vi "HumiditySensorInput.vi"(0 "FPGA I/O In":refnum<k21>="ConnectorA/DIO4") -> (4 "Temperature (°C)":fxp<+,16,7> format="%.11g", 6 "Humidity (%)":fxp<+/-,18,8> format="%.12g", 15 "error out":errorcluster)   [LabVIEW 2015, in "DHT22 (FPGA).lvlib"]
doc: "Read Temperature and Humidity from DHT11 Sensor.\n\n\nError Codes\n========\n\nError -8001: Checksum Error\nError- 8002: Timeout Error"
uses:
  DHT22 (FPGA).lvlib
  Command.ctl
  <vilib>/Platform/TimedLoop/XDataNode/timing_clust.ctl
  <vilib>/Platform/TimedLoop/XDataNode/nitl_modes.ctl
  <vilib>/Platform/TimedLoop/XDataNode/wakeup.ctl
  <vilib>/rvi/Emulation/niFpgaGetClockAttributes.vi
  <vilib>/rvi/Emulation/niFpgaSctlEmulationGetInTimedLoop.vi
  <vilib>/rvi/Emulation/niFpgaEmulationReportErrorSimple.vi
  <vilib>/rvi/Emulation/niFpgaProcessEmulError.vi
  <vilib>/rvi/Emulation/niFpgaCriticalErrorInLSC.vi
  <vilib>/rvi/eio/common/nirviEmuTemplateMethod_errors.vi
  <vilib>/Platform/TimedLoop/XDataNode/XDataNode.xnode
  <vilib>/eio/EIOMethodNode/EIOMethodNode.xnode
  <vilib>/eio/EIONode/EIONode.xnode
  <vilib>/Platform/TimedLoop/XDataNode/XDNodeRunTimeDep.lvlib
panel:
  in  "STOP Reading Inputs":bool
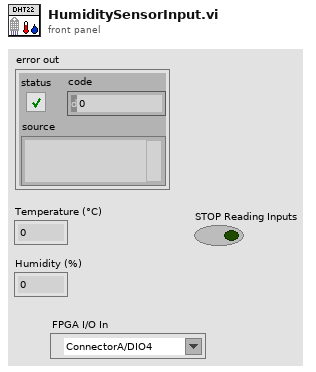
[diagram p1: front panel]
types:
  T1 = typedef "DHT22 (FPGA).lvlib/Command.ctl" = enum16{"Send Start Signal", "Wait Low", "Host Pulls Up", "Wait High", "Change to Read", "Wait for Sensor Response Signal Low", "Wait for Sensor Response Signal High", "Start Data Transmission", "Read Data", "Scale and Checksum", "Checksum Error", "Timeout Error"}
  T2 = typedef "XDNodeRunTimeDep.lvlib/timing_clust.ctl" = cluster{"Expected End [f-1]":u64, "Actual End [f-1]":u64, "Finished Late? [f-1]":bool, "Expected End [i-1]":u64, "Actual End [i-1]":u64, "Finished Late? [i-1]":bool, "Expected Start [i]":u64, "Actual Start [i]":u64, "Expected Start [f]":u64, "Actual Start [f]":u64, "Source Name":string, "Structure Name":string, "Period":i64, "Deadline":i64, "Offset":i64, "Start":i64, "Priority":i32, "Timeout":i32, "Mode":T3, "Wakeup Reason":T4, "Error":errorcluster, "Source Type":string, "Secondary Source Type":string, "Global End Time":u64, "Global Start Time":u64, "Frame Duration":u64, "Iteration Duration":u64, "Assigned CPU":i32, "I/O Scan Engine Mode":u32}
  T3 = typedef "XDNodeRunTimeDep.lvlib/nitl_modes.ctl" = enum32{"No Change", "Process missed periods, maintain original phase", "Discard missed periods, maintain original phase", "Process missed periods, ignore original phase", "Discard missed periods, ignore original phase"}
  T4 = typedef "XDNodeRunTimeDep.lvlib/wakeup.ctl" = enum32{"Normal", "Aborted", "Asynchronous wakeup", "Timing source error", "Timed loop error", "Timeout"}
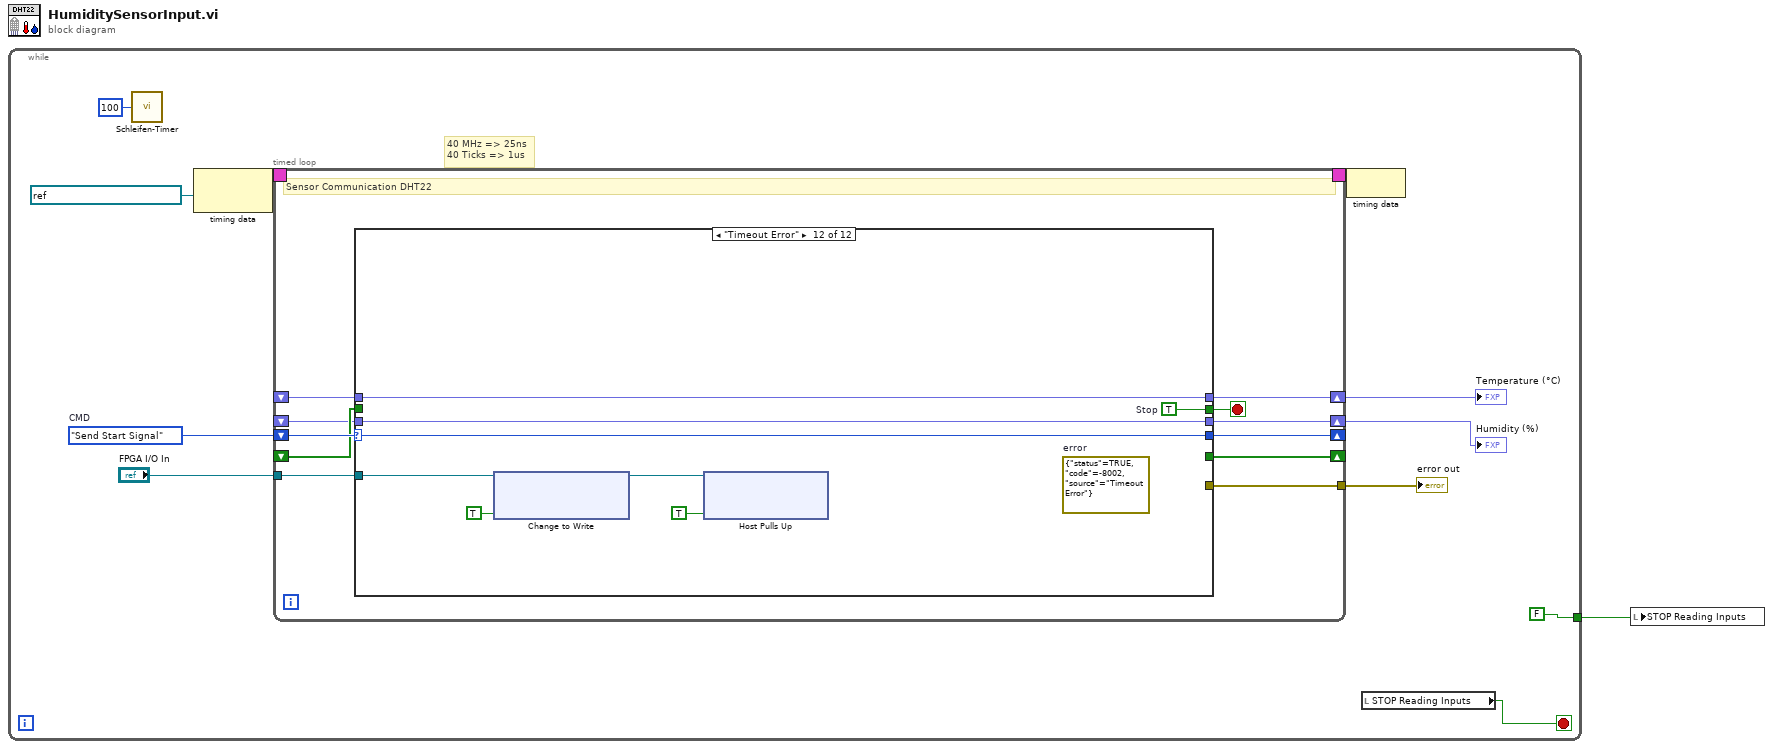
[diagram p0: block diagram]
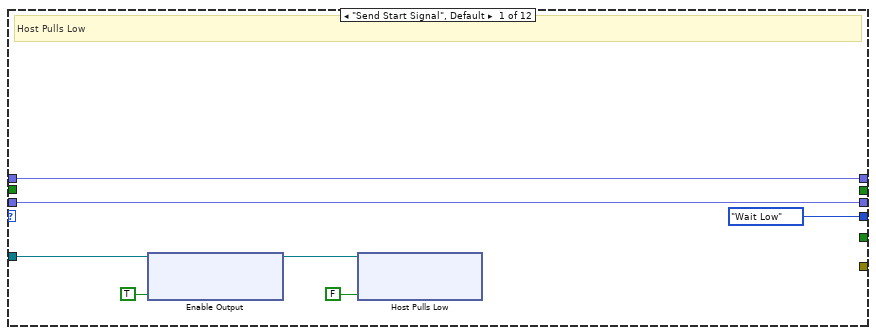
[diagram p2: hidden frame]
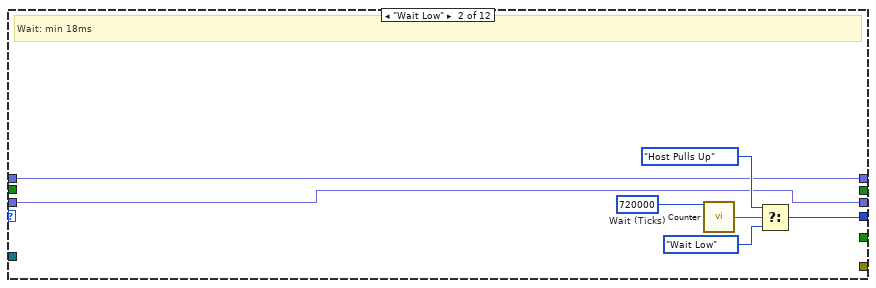
[diagram p3: hidden frame]
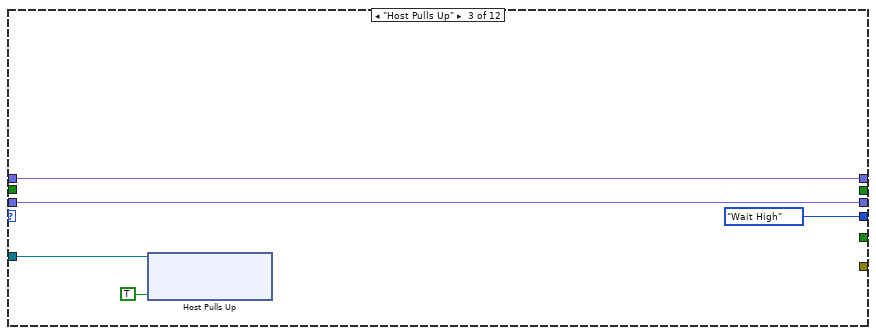
[diagram p4: hidden frame]
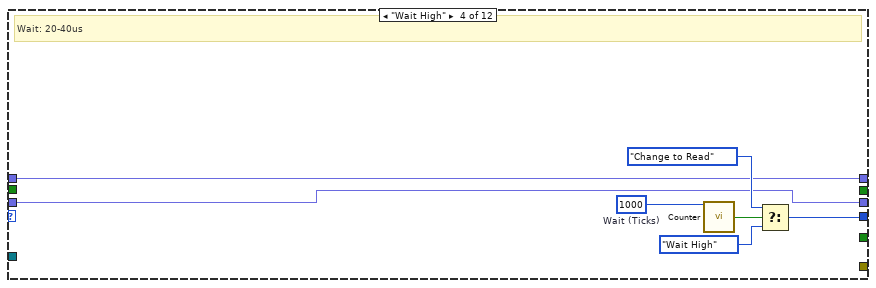
[diagram p5: hidden frame]
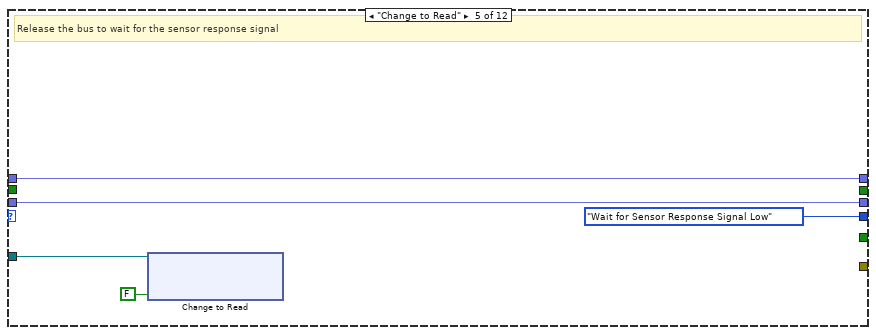
[diagram p6: hidden frame]
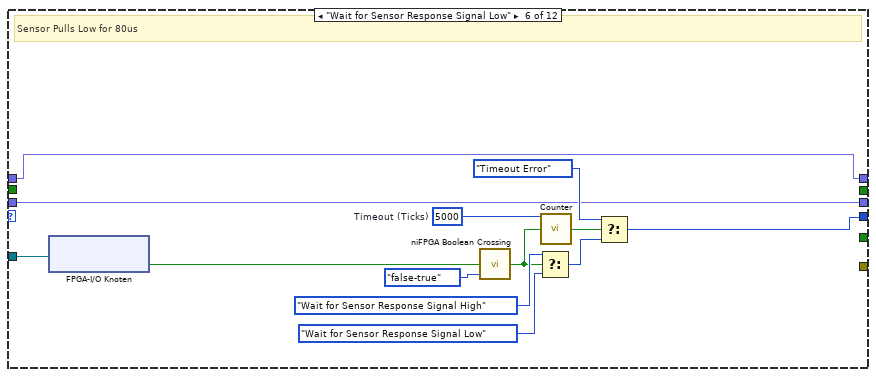
[diagram p7: hidden frame]
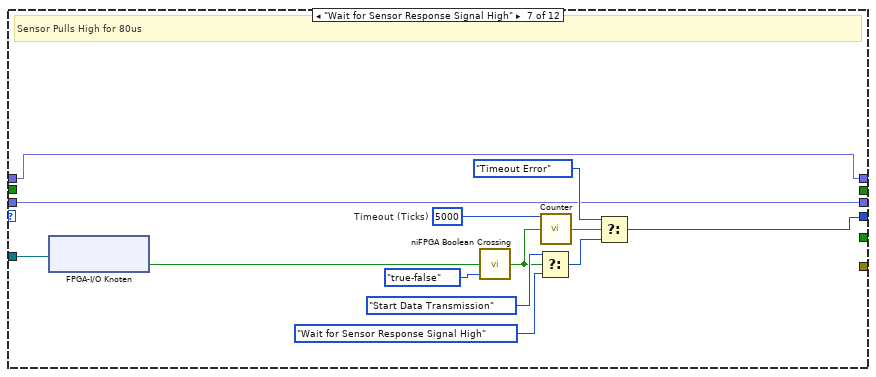
[diagram p8: hidden frame]
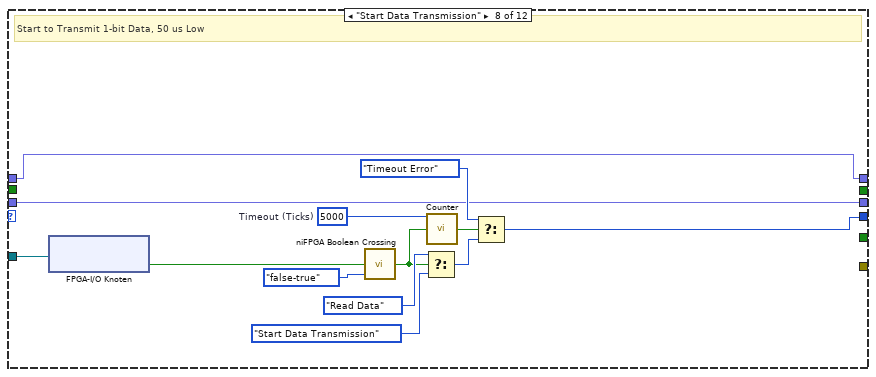
[diagram p9: hidden frame]
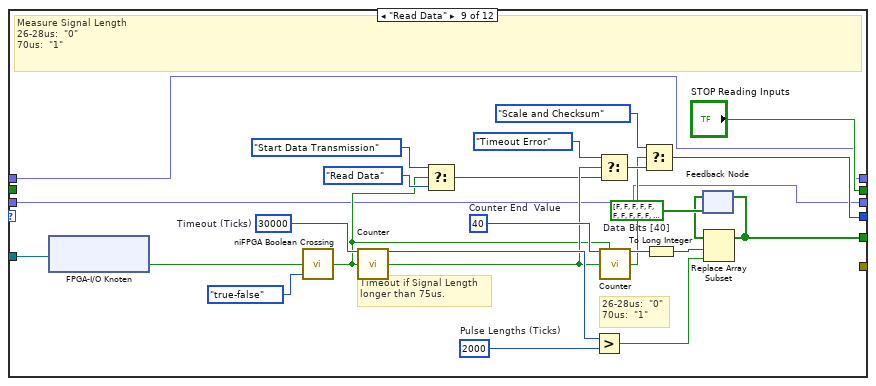
[diagram p10: hidden frame]
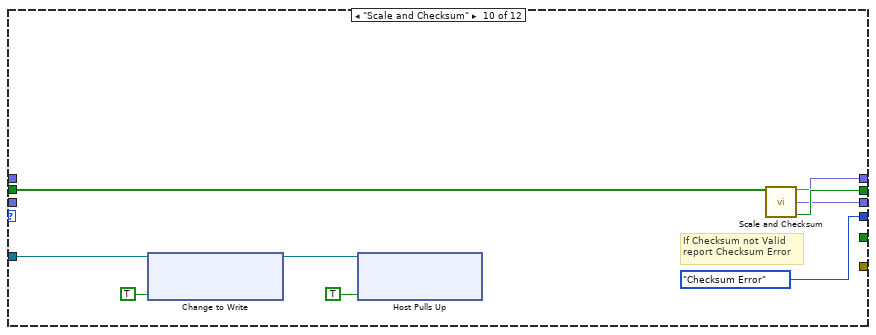
[diagram p11: hidden frame]
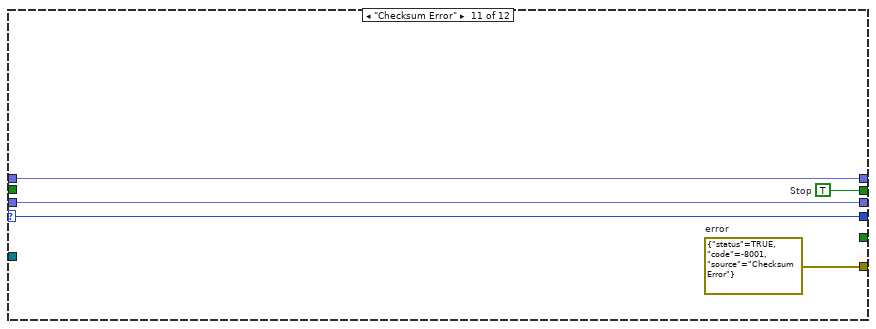
[diagram p12: hidden frame]
diagram:
  n1 = while {
    tunnel: [FALSE] -> w1
    stop <- w3 stop-if-true
    w10 = Command."Send Start Signal"  # CMD
    # "40 MHz => 25ns\n40 Ticks => 1us"
    n2 = call "Schleifen-Timer"("Count(mSec)"=u32 100) -> ()  [unwired: 1 out]
    n3 = node-c288(refnum<k21> "40 MHz Onboard Clock" ("Source Name")) -> (w12:T2)
    n4 = timed-loop {
      timing: w12 -> [_]
      timing-out: [_] -> w11
      shift-right: [w21] -> _
      shift-left: w10 -> [w23]
      tunnel: "FPGA I/O In" -> [w22]
      shift-right: [w19] -> _
      shift-left: _ -> [w18]
      tunnel: [w15] -> w6
      shift-right: [w17] -> w8
      shift-left: _ -> [w14]
      shift-right: [w16] -> w7
      shift-left: _ -> [w13]
      stop <- w20 stop-if-true
      # "Sensor Communication DHT22"
      n5 = case shown="\"Timeout Error\"" w23 {
        selector: w23 -> [_ _ _ _ _ _ _ _ _ _ w132 w140]
        tunnel: w22 -> [w29 _ w41 _ w53 w67 w80 w93 w119 w125 _ w136]
        tunnel: [Command."Wait Low" ("CMD") w35 Command."Wait High" ("CMD") w45 Command."Wait for Sensor Response Signal Low" ("CMD") w61 w74 w87 w100 Command."Checksum Error" ("CMD") w132 w140] -> w21
        tunnel: [_ _ _ _ _ _ _ _ "STOP Reading Inputs" w123 w133 w141] -> w20
        tunnel: [_ _ _ _ _ _ _ _ w98 _ _ _] -> w19
        tunnel: w18 -> [_ _ _ _ _ _ _ _ _ w124 _ _]
        tunnel: [w25 w31 w38 w43 w50 w55 w68 w81 w94 w121 w129 w134] -> w17
        tunnel: [w24 w32 w39 w44 w51 w56 w69 w82 w95 w120 w130 w135] -> w16
        tunnel: [_ _ _ _ _ _ _ _ _ _ w131 _] -> w15
        tunnel: w14 -> [w25 w31 w38 w43 w50 w55 w68 w81 w94 _ w129 w134]
        tunnel: w13 -> [w24 w32 w39 w44 w51 w56 w69 w82 w95 _ w130 w135]
        frame "Send Start Signal", Default {
          # "Host Pulls Low"
          n6 = xnode "Enable Output"("FPGA I/O In"=w29, "Enable"=TRUE ("Data")) -> ("FPGA I/O Out"=w27:refnum<k21>)
          n7 = xnode "Host Pulls Low"("FPGA I/O In"=w27, "Data"=FALSE ("Enable")) -> ()  [unwired: 1 out]
        }
        frame "Wait Low" {
          w37 = u32 720000  # Wait (Ticks)
          # "Wait: min 18ms"
          n8 = call "Counter.vi"("Counter End  Value"=w37) -> ("End Reached"=w33:bool)  [unwired: 13 in, 1 out]
          n9 = Select(t=Command."Host Pulls Up" ("CMD"), s=w33, f=Command."Wait Low" ("CMD")) -> (s? t:f=w35:T1)
        }
        frame "Host Pulls Up" {
          n10 = xnode "Host Pulls Up"("FPGA I/O In"=w41, "Data"=TRUE ("Enable")) -> ()  [unwired: 1 out]
        }
        frame "Wait High" {
          w49 = u32 1000  # Wait (Ticks)
          # "Wait: 20-40us"
          n11 = call "Counter.vi"("Counter End  Value"=w49) -> ("End Reached"=w46:bool)  [unwired: 13 in, 1 out]
          n12 = Select(t=Command."Change to Read" ("CMD"), s=w46, f=Command."Wait High" ("CMD")) -> (s? t:f=w45:T1)
        }
        frame "Change to Read" {
          # "Release the bus to wait for the sensor response signal"
          n13 = xnode "Change to Read"("FPGA I/O In"=w53, "Enable"=FALSE ("Data")) -> ()  [unwired: 1 out]
        }
        frame "Wait for Sensor Response Signal Low" {
          w66 = u32 5000  # Timeout (Ticks)
          # "Sensor Pulls Low for 80us"
          n14 = xnode "FPGA-I/O Knoten"("FPGA-I/O (Eingang)"=w67) -> ("I/O-Objekt"=w62:bool)  [unwired: 1 out]
          n15 = call <vilib>:"niFPGA Boolean Crossing.vi"("input"=w62, "direction"=enum8{"either", "false-true", "true-false"}."false-true") -> ("crossing"=w57:bool)  [unwired: 7 in]
          n16 = Select(t=Command."Wait for Sensor Response Signal High" ("CMD"), s=w57, f=Command."Wait for Sensor Response Signal Low" ("CMD")) -> (s? t:f=w60:T1)
          n17 = call "Counter.vi"("Counter End  Value"=w66, "Reset"=w57) -> ("End Reached"=w58:bool)  [unwired: 12 in, 1 out]
          n18 = Select(t=Command."Timeout Error", s=w58, f=w60) -> (s? t:f=w61:T1)
        }
        frame "Wait for Sensor Response Signal High" {
          w79 = u32 5000  # Timeout (Ticks)
          # "Sensor Pulls High for 80us"
          n19 = xnode "FPGA-I/O Knoten"("FPGA-I/O (Eingang)"=w80) -> ("I/O-Objekt"=w75:bool)  [unwired: 1 out]
          n20 = call <vilib>:"niFPGA Boolean Crossing.vi"("input"=w75, "direction"=enum8{"either", "false-true", "true-false"}."true-false") -> ("crossing"=w70:bool)  [unwired: 7 in]
          n21 = Select(t=Command."Start Data Transmission" ("CMD"), s=w70, f=Command."Wait for Sensor Response Signal High" ("CMD")) -> (s? t:f=w73:T1)
          n22 = call "Counter.vi"("Counter End  Value"=w79, "Reset"=w70) -> ("End Reached"=w71:bool)  [unwired: 12 in, 1 out]
          n23 = Select(t=Command."Timeout Error", s=w71, f=w73) -> (s? t:f=w74:T1)
        }
        frame "Start Data Transmission" {
          w92 = u32 5000  # Timeout (Ticks)
          # "Start to Transmit 1-bit Data, 50 us Low"
          n24 = xnode "FPGA-I/O Knoten"("FPGA-I/O (Eingang)"=w93) -> ("I/O-Objekt"=w88:bool)  [unwired: 1 out]
          n25 = call <vilib>:"niFPGA Boolean Crossing.vi"("input"=w88, "direction"=enum8{"either", "false-true", "true-false"}."false-true") -> ("crossing"=w83:bool)  [unwired: 7 in]
          n26 = Select(t=Command."Read Data" ("CMD"), s=w83, f=Command."Start Data Transmission" ("CMD")) -> (s? t:f=w86:T1)
          n27 = call "Counter.vi"("Counter End  Value"=w92, "Reset"=w83) -> ("End Reached"=w84:bool)  [unwired: 12 in, 1 out]
          n28 = Select(t=Command."Timeout Error", s=w84, f=w86) -> (s? t:f=w87:T1)
        }
        frame "Read Data" {
          w118 = u32 30000  # Timeout (Ticks)
          w112 = u32 2000  # Pulse Lengths (Ticks)
          w106 = u32 40  # Counter End  Value
          w110 = bool[] [FALSE, FALSE, FALSE, FALSE, FALSE, FALSE, FALSE, FALSE, FALSE, FALSE, FALSE, FALSE, FALSE, FALSE, FALSE, FALSE, FALSE, FALSE, FALSE, FALSE, FALSE, FALSE, FALSE, FALSE, FALSE, FALSE, FALSE, FALSE, FALSE, FALSE, FALSE, FALSE, FALSE, FALSE, FALSE, FALSE, FALSE, FALSE, FALSE, FALSE]  # Data Bits [40]
          # "26-28us:  \"0\"\n70us:  \"1\""
          # "Timeout if Signal Length\nlonger than 75us."
          # "Measure Signal Length\n26-28us:  \"0\"\n70us:  \"1\""
          n29 = xnode "FPGA-I/O Knoten"("FPGA-I/O (Eingang)"=w119) -> ("I/O-Objekt"=w114:bool)  [unwired: 1 out]
          n30 = call <vilib>:"niFPGA Boolean Crossing.vi"("input"=w114, "direction"=enum8{"either", "false-true", "true-false"}."true-false") -> ("crossing"=w103:bool)  [unwired: 7 in]
          n31 = call "Counter.vi"("Counter End  Value"=w118, "Reset"=w103) -> ("Counter Value"=w111:u32, "End Reached"=w104:bool)  [unwired: 12 in]
          n32 = Select(t=Command."Start Data Transmission" ("CMD"), s=w103, f=Command."Read Data" ("CMD")) -> (s? t:f=w102:T1)
          n33 = Greater?(x=w111, y=w112) -> (0:w107:bool)
          n34 = Select(t=Command."Timeout Error", s=w104, f=w102) -> (s? t:f=w99:T1)
          n35 = call "Counter.vi"("Counter End  Value"=w106, "Input Valid"=w103, "Reset"=w104) -> ("Counter Value"=w105:u32, "End Reached"=w97:bool)  [unwired: 11 in]
          n36 = Select(t=Command."Scale and Checksum", s=w97, f=w99) -> (s? t:f=w100:T1)
          n37 = To Long Integer(number=w105) -> (32bit integer=w108:i32)
          n38 = feedback #1(w110) -> (w109:bool[])
          n39 = Replace Array Subset(array=w109, new element=w107, index=w108) -> (w98:bool[])
          n40 = feedback-in #1(w98) -> ()
        }
        frame "Scale and Checksum" {
          # "If Checksum not Valid\nreport Checksum Error"
          n41 = xnode "Change to Write"("FPGA I/O In"=w125, "Enable"=TRUE ("Data")) -> ("FPGA I/O Out"=w126:refnum<k21>)
          n42 = xnode "Host Pulls Up"("FPGA I/O In"=w126, "Data"=TRUE ("Enable")) -> ()  [unwired: 1 out]
          n43 = call "Scale and Checksum.vi"("Raw Data"=w124) -> ("Temperature (°C)"=w121:fxp<+,16,7>, "Humidity (%)"=w120:fxp<+/-,18,8>, "Valid?"=w123:bool)  [unwired: 12 in]
        }
        frame "Checksum Error" {
          w131 = errorcluster {"status"=TRUE, "code"=-8001, "source"="Checksum Error"}  # error
          w133 = TRUE  # Stop
        }
        frame "Timeout Error" {
          (unwired) errorcluster {"status"=TRUE, "code"=-8002, "source"="Timeout Error"}  # error
          w141 = TRUE  # Stop
          n44 = xnode "Change to Write"("FPGA I/O In"=w136, "Enable"=TRUE ("Data")) -> ("FPGA I/O Out"=w137:refnum<k21>)
          n45 = xnode "Host Pulls Up"("FPGA I/O In"=w137, "Data"=TRUE ("Enable")) -> ()  [unwired: 1 out]
        }
      }
    }
    "Temperature (°C)" <- w8
    "Humidity (%)" <- w7
    "error out" <- w6
    n46 = node-c288(w11) -> ()
    n47 = local read "STOP Reading Inputs"() -> (w3:bool)
  }
  n48 = local write "STOP Reading Inputs"(w1) -> ()
